vi "estiDofByZTAAC.vi"() -> ()   [LabVIEW 2016]
uses:
  ZTAAC/ZTAAC.lvclass
  StrictDef/FilterType.ctl
  CamRot/CamRot.lvclass
  StrictDef/InstName.ctl
  StrictDef/DofGroup.ctl
  OfcFunc.lvlib
panel:
  in  "ZTAAC Configuration":T2={"Config Dir"=path "/home/ttsai/Documents/github/ts_tcs_ofc/configData", "Inst Name"=enum."lsst", "OptStateEsti Config File Name"="pinv.esti", "Mapping File Name"="sensorNameToFieldIdx.txt", "Wavelength Table"="effWaveLength.txt", "Intrinc Zk File Name"="intrinsic_zn", "y2 Corection File Name"="y2.txt", "Index DOF File Name"="idxDOF.txt", "OptCtrl Config File Name"="optiPSSN_x00.ctrl", "State 0 File Name"="state0inDof.txt", "Weighting File Name"="imgQualWgt.txt", "PSSN Alpha File Name"="pssn_alpha.txt", "Authority Files"={"Rigid Body Stroke File"="rbStroke.txt", "M1M3 Subsystem"={"Mirror"="M1M3", "Actuatro Force File"="M1M3_1um_156_force.txt"}, "M2 Subsystem"={"Mirror"="M2", "Actuatro Force File"="M2_1um_force.DAT"}, "Num of Bending Mode"=20}, "Sensor Id to Name File Name"="sensorIdToName.txt", "Truncation Threshold"=0.0001, "Default Gain"=0.7, "FWHM Threshold (arcsec)"=0.2}
  in  "Sensor Id":i32[](array[numeric])=[198, 31, 2, 169, -1]
  out "Agg. Uk of M2 Bend":dbl[](array[numeric])
  out "Agg. Uk of M1M3 Bend":dbl[](array[numeric])
  out "Agg. Uk of Camera Hex Pos":dbl[](array[numeric])
  out "Agg. Uk of M2 Hex Pos":dbl[](array[numeric])
  in  "Rotation Angle in Deg":dbl
  in  "CamRot.lvclass":refnum<class "CamRot.lvclass">
  in  "Filter Type":T3
  out "Sensor Name":string[](array[string])=["R:4,4 S:0,0", "R:0,4 S:2,0", "R:0,0 S:2,2", "R:4,0 S:0,2"]
  in  "Wfs Err Data":path=path "/home/ttsai/Documents/github/ts_tcs_ofc/testData/lsst_wfs_error_iter0.z4c"
  in  "Gain":dbl=1.0
  in  "ZTAAC.lvclass":refnum<class "ZTAAC.lvclass">
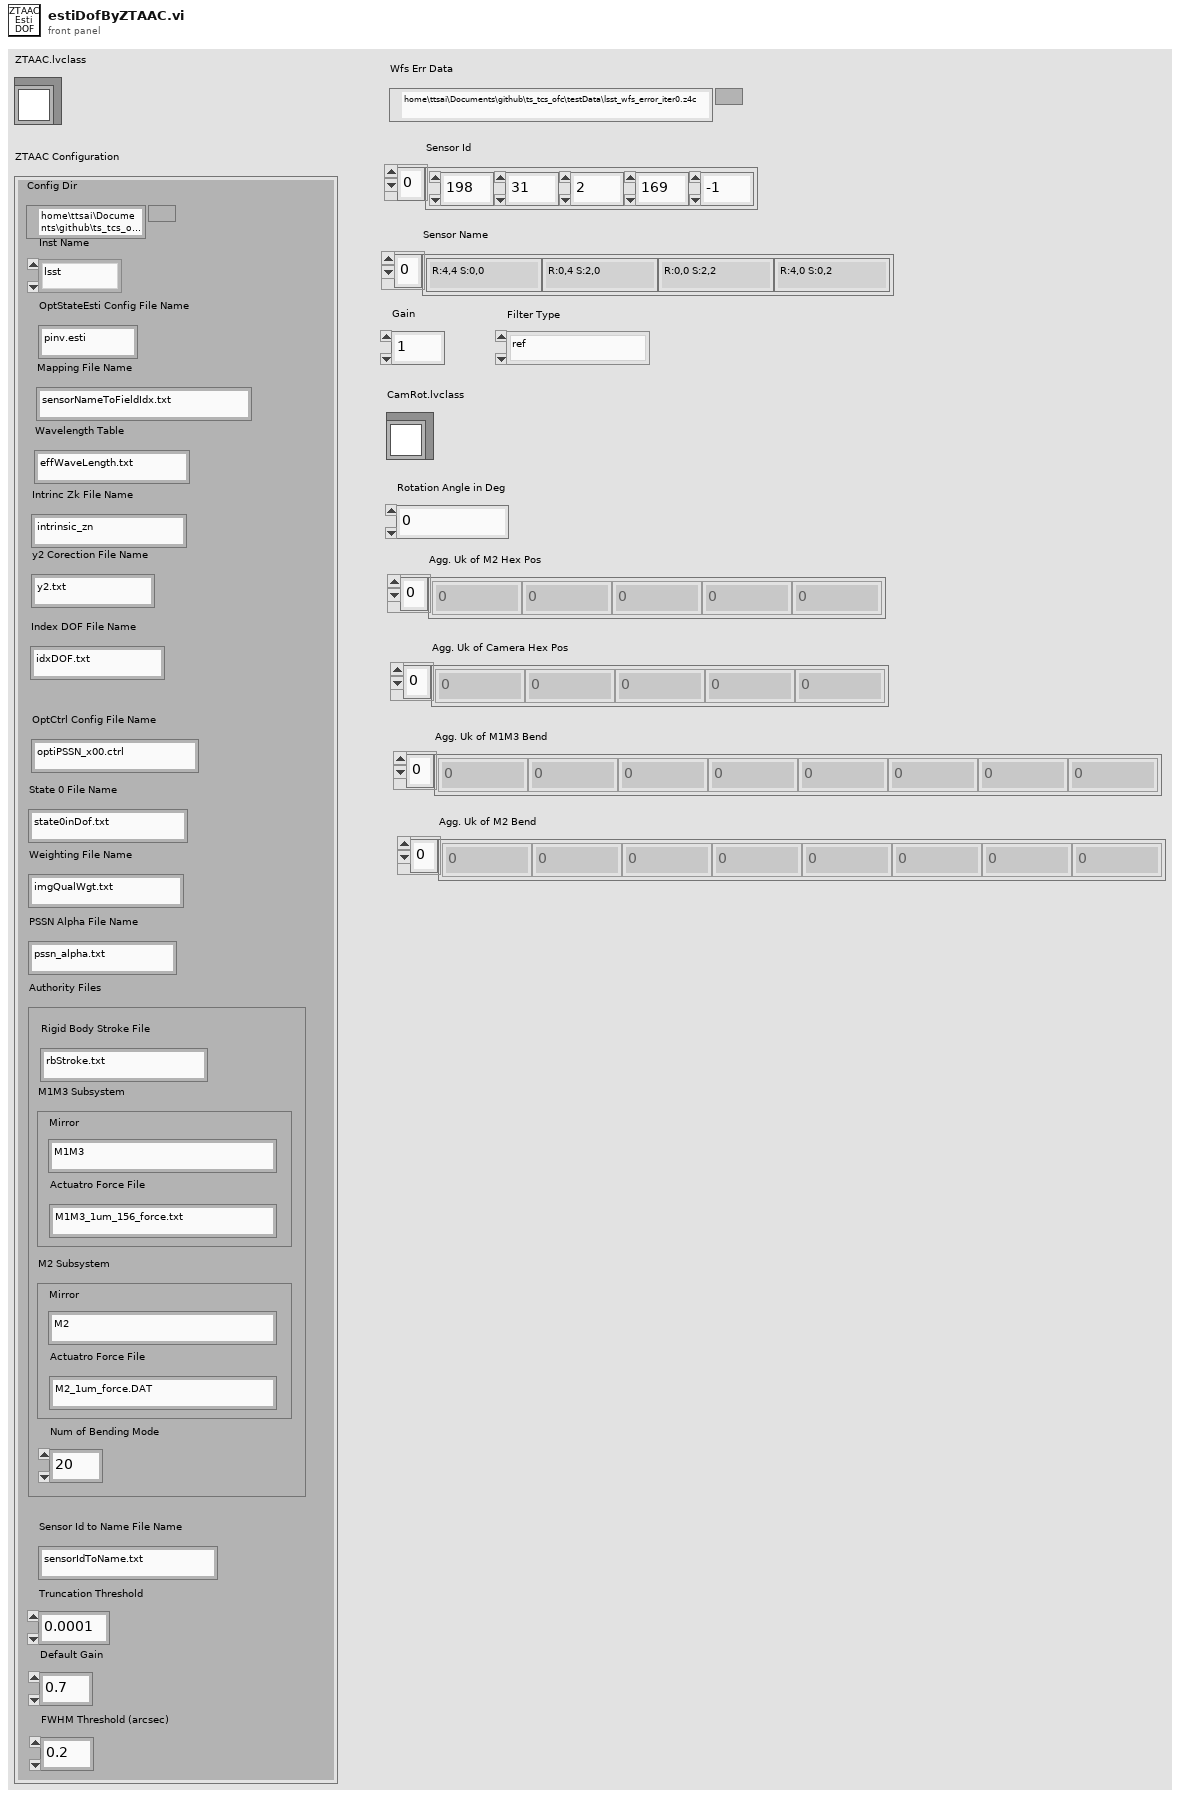
[diagram p1: front panel]
types:
  T1 = typedef "OfcFunc.lvlib/InstName.ctl" = enum16{"lsst", "comcam"}
  T2 = cluster{"Config Dir":path, "Inst Name":T1, "OptStateEsti Config File Name":string, "Mapping File Name":string, "Wavelength Table":string, "Intrinc Zk File Name":string, "y2 Corection File Name":string, "Index DOF File Name":string, "OptCtrl Config File Name":string, "State 0 File Name":string, "Weighting File Name":string, "PSSN Alpha File Name":string, "Authority Files":cluster{"Rigid Body Stroke File":string, "M1M3 Subsystem":cluster{"Mirror":string, "Actuatro Force File":string}, "M2 Subsystem":cluster{"Mirror":string, "Actuatro Force File":string}, "Num of Bending Mode":i32}, "Sensor Id to Name File Name":string, "Truncation Threshold":dbl, "Default Gain":dbl, "FWHM Threshold (arcsec)":dbl}
  T3 = typedef "OfcFunc.lvlib/FilterType.ctl" = enum16{"ref", "u", "g", "r", "i", "z", "y"}
  T4 = typedef "OfcFunc.lvlib/DofGroup.ctl" = enum16{"M2 Hex Pos", "Cam Hex Pos", "M1M3 Bend", "M2 Bend"}
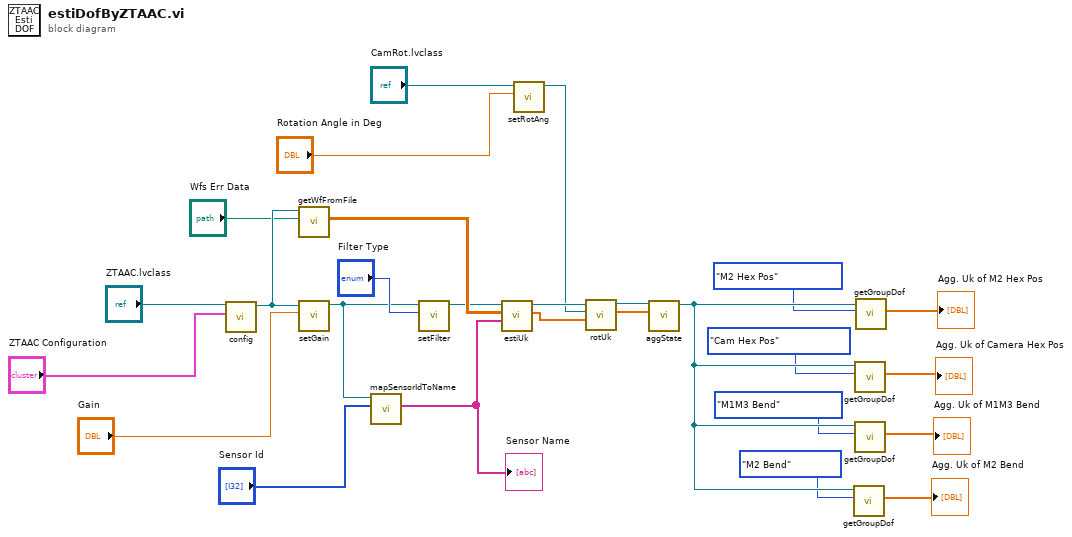
[diagram p0: block diagram]
diagram:
  n1 = call "config.vi"("ZTAAC Configuration"="ZTAAC Configuration", "ZTAAC in"="ZTAAC.lvclass") -> ("ZTAAC out"=w25:refnum<class "ZTAAC.lvclass">)  [unwired: 8 in, 1 out]
  n2 = call "getWfFromFile.vi"("Wfs Err Data"="Wfs Err Data", "ZTAAC in"=w25) -> ("Wavefront Error"=w6:dbl[][])  [unwired: 7 in, 2 out]
  n3 = call "setGain.vi"("Gain"="Gain", "ZTAAC in"=w25) -> ("ZTAAC out"=w4:refnum<class "ZTAAC.lvclass">)  [unwired: 8 in, 1 out]
  n4 = call "mapSensorIdToName.vi"("Sensor Id"="Sensor Id", "ZTAAC in"=w4) -> ("Sensor Name"=w2:string[])  [unwired: 6 in, 3 out]
  "Sensor Name" <- w2
  n5 = call "setFilter.vi"("Filter Type"="Filter Type", "ZTAAC in"=w4) -> ("ZTAAC out"=w5:refnum<class "ZTAAC.lvclass">)  [unwired: 8 in, 1 out]
  n6 = call "estiUk.vi"("Sensor Name"=w2, "Wavefront Error"=w6, "ZTAAC in"=w5) -> ("uk Array"=w15:dbl[], "ZTAAC out"=w16:refnum<class "ZTAAC.lvclass">)  [unwired: 6 in, 1 out]
  n7 = call "setRotAng.vi"("Rotation Angle in Deg"="Rotation Angle in Deg", "CamRot in"="CamRot.lvclass") -> ("CamRot out"=w12:refnum<class "CamRot.lvclass">)  [unwired: 8 in, 1 out]
  n8 = call "rotUk.vi"("uk Array"=w15, "CamRot in"=w12, "ZTAAC in"=w16) -> ("Rotated uk Array"=w14:dbl[], "ZTAAC out"=w13:refnum<class "ZTAAC.lvclass">)  [unwired: 6 in, 1 out]
  n9 = call "aggState.vi"("State in DOF"=w14, "ZTAAC in"=w13) -> ("ZTAAC out"=w23:refnum<class "ZTAAC.lvclass">)  [unwired: 8 in, 1 out]
  n10 = call "getGroupDof.vi"("DOF Group"=DofGroup."M2 Bend", "ZTAAC in"=w23) -> ("DOF"=→"Agg. Uk of M2 Bend":dbl[])  [unwired: 7 in, 2 out]
  n11 = call "getGroupDof.vi"("DOF Group"=DofGroup."Cam Hex Pos", "ZTAAC in"=w23) -> ("DOF"=→"Agg. Uk of Camera Hex Pos":dbl[])  [unwired: 7 in, 2 out]
  n12 = call "getGroupDof.vi"("DOF Group"=DofGroup."M1M3 Bend", "ZTAAC in"=w23) -> ("DOF"=→"Agg. Uk of M1M3 Bend":dbl[])  [unwired: 7 in, 2 out]
  n13 = call "getGroupDof.vi"("DOF Group"=DofGroup."M2 Hex Pos", "ZTAAC in"=w23) -> ("DOF"=→"Agg. Uk of M2 Hex Pos":dbl[])  [unwired: 7 in, 2 out]
